vi "sv_Build Even Angle Signal (N Channels).vi"(5 "# of ch":i32, 8 "samples/rev":dbl, 9 "offset":dbl, 10 "time stamps":dbl[](array[numeric]) format="%.2f", 11 "Data":dbl[][](array[numeric]) format="%.2f") -> (2 "even-angle position info":T1, 3 "even-angle signals":cluster{"r0":dbl, "dr":dbl, "Y":dbl[]}[](array[cluster]) {"r0" format="%.2p"; "dr" format="%.2p"; "Y" format="%.2f"})   [LabVIEW 2017, in "SoundVib_Resampling.lvlib"]
uses:
  <vilib>/addons/Sound and Vibration/Order Analysis/Resample Order Tracking/SoundVib_Resampling.lvlib
  <vilib>/addons/Sound and Vibration/Order Analysis/Misc/OAT Position Info.ctl
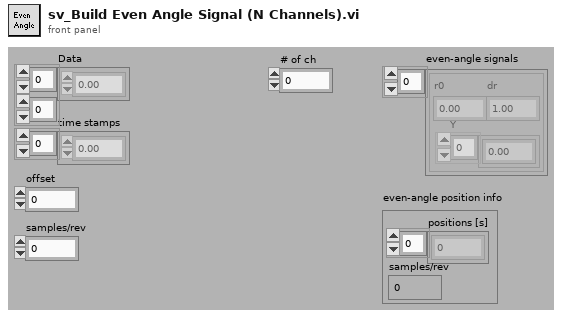
[diagram p1: front panel]
types:
  T1 = typedef "OAT Position Info.ctl" = cluster{"positions [s]":dbl[], "samples/rev":dbl}
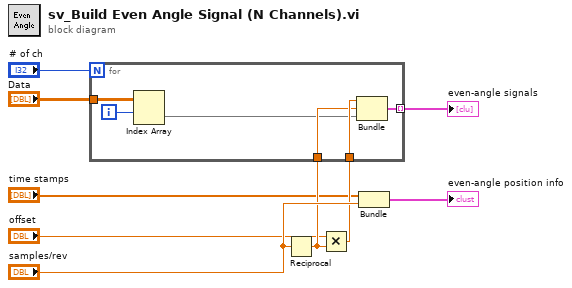
[diagram p0: block diagram]
diagram:
  n1 = Reciprocal(x="samples/rev") -> (1/x=w3:dbl)
  n2 = Multiply(x="offset", y=w3) -> (x*y=w4:dbl)
  n3 = for {
    N: "# of ch" -> [_]
    tunnel: w4 -> [w15]
    tunnel: w3 -> [w14]
    tunnel: [w13] -> w5 mode=indexing
    tunnel: "Data" -> [w12]
    i -> [w11]
    n4 = Index Array(array=w12, index (row)=w11) -> (element=w10:dbl[])  [unwired: 1 in]
    n5 = Bundle(w15, w14, "Data"=w10) -> (w13:cluster{dbl, dbl, "Data":dbl[]})  [unwired: 1 in]
  }
  "even-angle signals" <- w5
  n6 = Bundle("time stamps"="time stamps", "samples/rev"="samples/rev") -> (→"even-angle position info":cluster{"time stamps":dbl[], "samples/rev":dbl})  [unwired: 1 in]
